vi "Logging_Example.vi"() -> ()   [LabVIEW 2024]
uses:
  Stream/Writer/DETT/DETTWriter.lvclass
  C:/Git/JA/JQMH/RQMHCore/Stream/INetworkWriter/INetworkWriter.lvclass
  LogFormatter/Default/DefaultLogFormat.lvclass
  C:/Git/JA/JQMH/RQMHCore/ErrorReporting/LogFormatter/Interface/ILogFormatter.lvclass
  LogHandle/Event/EventLogHandle.lvclass/EventLogHandle.ctl
  Record/LogRecord.lvclass/LogRecord.ctl
  RQMHLogger/Logger.lvclass/Logger.ctl
  HandleHolder/HandleHolder.lvclass/HandleHolder.ctl
  LogHandle/Stream/StreamLogHandle.lvclass
  C:/Git/JA/JQMH/RQMHCore/ErrorReporting/LogHandle/Interface/LoggingHandle.lvclass
  Stream/ConsoleWriter/ConsoleWriter.lvclass
  LogHandle/SQLiteLogHandle/SQLiteLogHandle.lvclass
  LogHandle/Event/EventLogHandle.lvclass
  <vilib>/drjdpowell/SQLite Library/SQL Connection/Connection.lvclass
  Record/LogRecord.lvclass
  LogHandle/Interface/LoggingHandle.lvclass
  RQMHLogger/Logger.lvclass
  HandleHolder/HandleHolder.lvclass
  <vilib>/drjdpowell/SQLite Library/SQLite.lvlib
  <vilib>/drjdpowell/SQLite Library/SQL Connection/Open (string).vi
  <vilib>/drjdpowell/SQLite Library/SQL Connection/Execute SQL.vi
  Shared/Level.ctl
  Shared/LoggerShared.lvlib
panel:
  out "error out 2":errorcluster
  out "Result Set":string[][](table) caption="Result Set (from first statement with results)"
  in  "stop":bool
  out "error out":errorcluster
  out "Level":T1
  out "Source":string
  out "Message":string
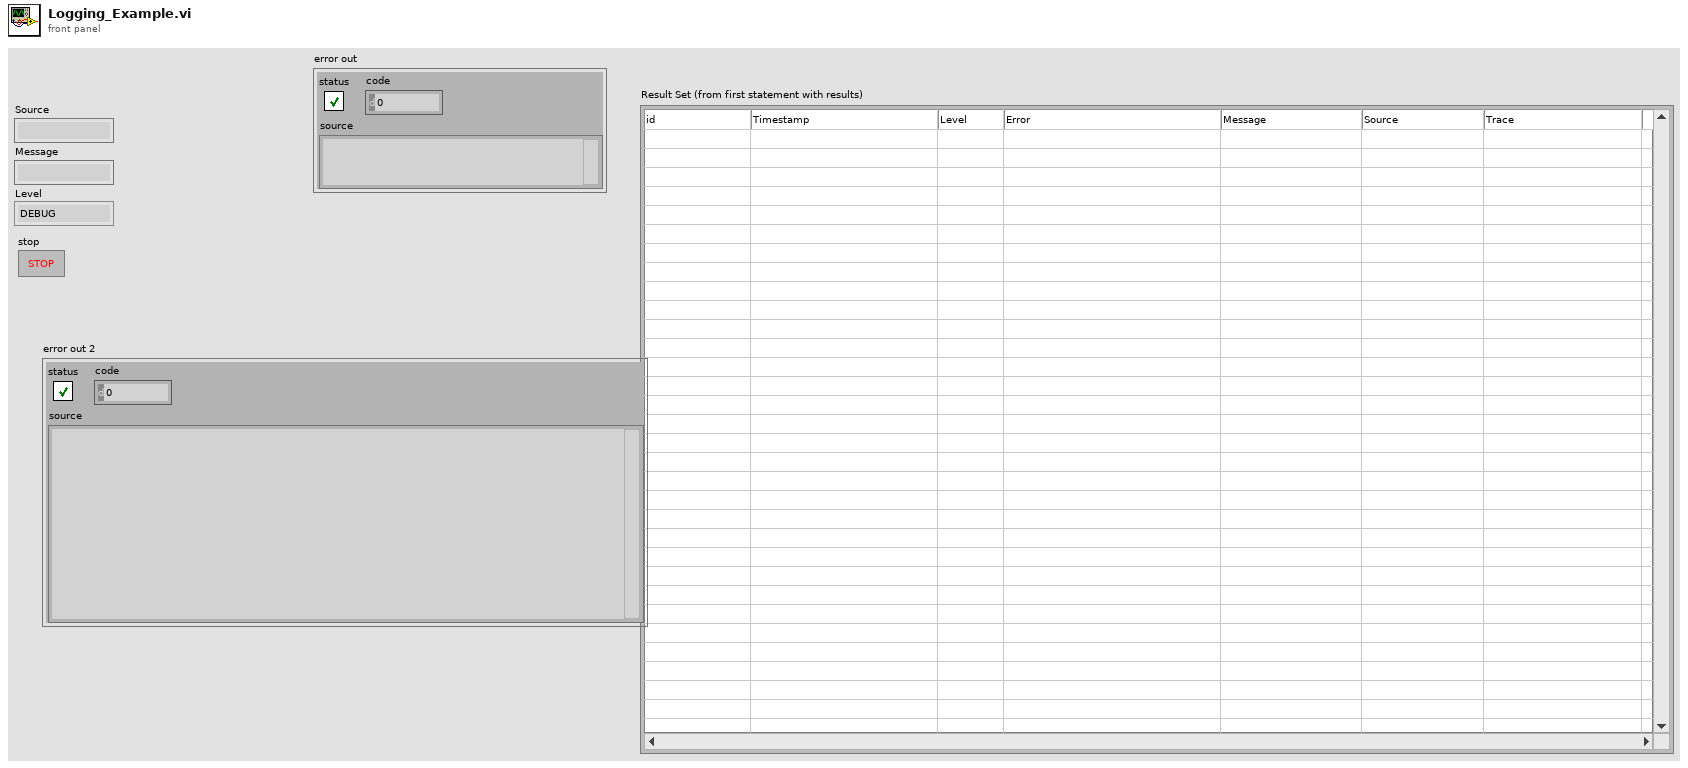
[diagram p1: front panel]
types:
  T1 = typedef "LoggerShared.lvlib/Level.ctl" = enum16{"DEBUG", "INFO", "WARNING", "ERROR", "CRITICAL"}
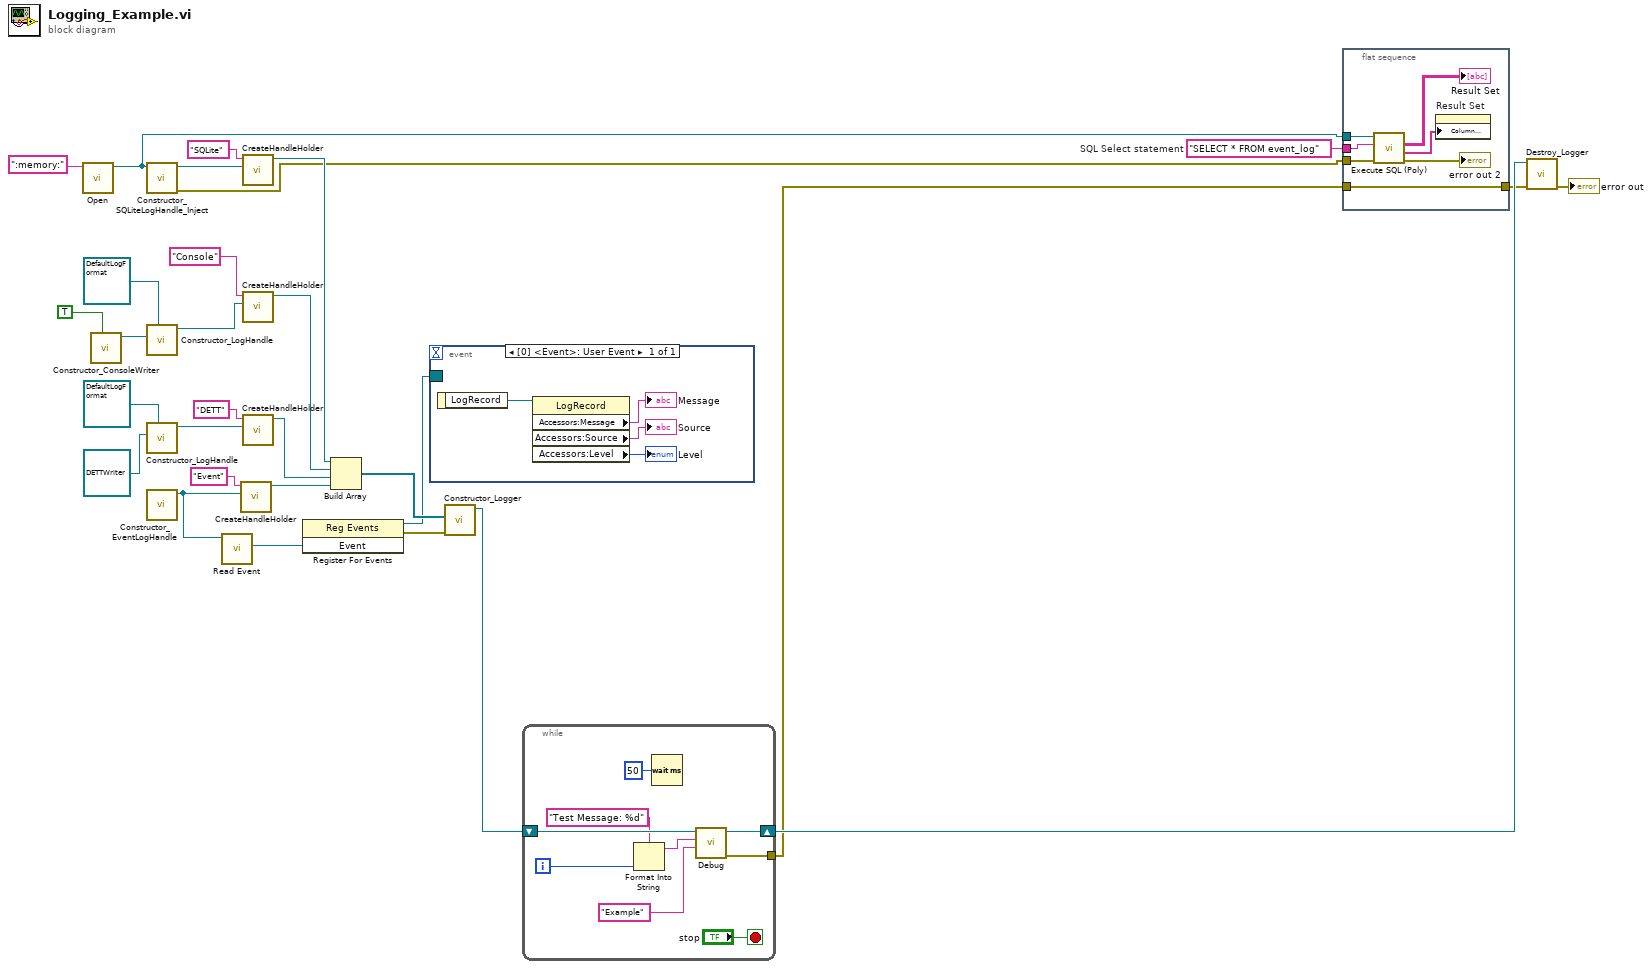
[diagram p0: block diagram]
diagram:
  w7 = "SELECT * FROM event_log"  # SQL Select statement
  (unwired) TRUE ("Autoshow? (f)")
  (unwired) refnum<class "DefaultLogFormat.lvclass"> refnum ("DefaultLogFormat.lvclass")
  n1 = call-poly <vilib>:"Open.vi"("db file"=":memory:") -> ("SQLite Connection"=w6:refnum<class "Connection.lvclass">)  [unwired: 9 in, 1 out]
  n2 = call "Constructor_ConsoleWriter.vi"("Autoshow? (f)"=TRUE) -> ("ConsoleWriter out"=w14:refnum<class "ConsoleWriter.lvclass">)  [unwired: 9 in, 1 out]
  n3 = call "Constructor_SQLiteLogHandle_Inject.vi"("Connection in"=w6) -> ("error out"=w5:errorcluster, "SQLiteLogHandle out"=w10:refnum<class "SQLiteLogHandle.lvclass">)  [unwired: 9 in]
  n4 = call "Constructor_LogHandle.vi"("Formatter"=refnum<class "DefaultLogFormat.lvclass"> refnum ("DefaultLogFormat.lvclass"), "INetworkWriter"=w14) -> ("FileHandler out"=w18:refnum<class "StreamLogHandle.lvclass">)  [unwired: 8 in, 1 out]
  n5 = call "Constructor_LogHandle.vi"("Formatter"=refnum<class "DefaultLogFormat.lvclass"> refnum ("DefaultLogFormat.lvclass"), "INetworkWriter"=refnum<class "DETTWriter.lvclass"> refnum ("DETTWriter.lvclass")) -> ("FileHandler out"=w20:refnum<class "StreamLogHandle.lvclass">)  [unwired: 8 in, 1 out]
  n6 = call "Constructor_EventLogHandle.vi"() -> ("EventHandle"=w27:refnum<class "EventLogHandle.lvclass">)  [unwired: 10 in, 1 out]
  n7 = call "Read Event.vi"("EventLogHandle in"=w27) -> ("Event"=w26:refnum<user-event>)  [unwired: 8 in, 2 out]
  n8 = call "CreateHandleHolder.vi"("Handle"=w27, "Name"="Event") -> ("HandleHolder out"=w29:refnum<class "HandleHolder.lvclass">)  [unwired: 9 in]
  n9 = call "CreateHandleHolder.vi"("Handle"=w10, "Name"="SQLite") -> ("HandleHolder out"=w8:refnum<class "HandleHolder.lvclass">)  [unwired: 9 in]
  n10 = call "CreateHandleHolder.vi"("Handle"=w18, "Name"="Console") -> ("HandleHolder out"=w15:refnum<class "HandleHolder.lvclass">)  [unwired: 9 in]
  n11 = call "CreateHandleHolder.vi"("Handle"=w20, "Name"="DETT") -> ("HandleHolder out"=w22:refnum<class "HandleHolder.lvclass">)  [unwired: 9 in]
  n12 = register-events(w26) -> (reference out=w25:refnum<event-registration>, error out=w24:errorcluster)  [unwired: 2 in]
  n13 = Build Array(w8, w15, w22, w29) -> (w28:refnum<class "HandleHolder.lvclass">[])
  n14 = event shown="[0] <Event>: User Event" {
    selector: w25 -> [_]
    dyn-events: _ -> [_]
    timeout: _ -> [_]
    event User Event {
      n15 = event-data() -> ("LogRecord"=w34:refnum<class "LogRecord.lvclass">)  [unwired: 1 in]
      n16 = property class="LogRecord"(reference=w34) -> ("Accessors:Message"=→"Message":string, "Accessors:Source"=→"Source":string, "Accessors:Level"=→"Level":T1)  [unwired: 1 in, 2 out]
    }
  }
  n17 = call "Constructor_Logger.vi"("error in (no error)"=w24, "Handles"=w28) -> ("RQMHLogger out"=w12:refnum<class "Logger.lvclass">)  [unwired: 8 in, 1 out]
  n18 = while {
    tunnel: [w40] -> w1
    shift-right: [w35] -> w4
    shift-left: w12 -> [w41]
    i -> [w37]
    stop <- "stop" stop-if-true
    n19 = Format Into String(format string="Test Message: %d" ("Message"), w37) -> (resulting string=w38:string)  [unwired: 2 in, 1 out]
    n20 = Wait (ms)(milliseconds to wait=u32 50) -> ()  [unwired: 1 out]
    n21 = call "Debug.vi"("Source"="Example", "Message"=w38, "RQMHLogger in"=w41) -> ("error out"=w40:errorcluster, "RQMHLogger out"=w35:refnum<class "Logger.lvclass">)  [unwired: 7 in]
  }
  n22 = flat-sequence {
    tunnel: w7 -> [w50]
    tunnel: w6 -> [w49]
    tunnel: w5 -> [w48]
    tunnel: [w44] -> w2
    tunnel: w1 -> [w44]
    frame #0 {
      n23 = call-poly <vilib>:"Execute SQL (Poly).vi"("error in (no error)"=w48, "SQL"=w50, "SQLite Connection in"=w49) -> ("error out"=→"error out 2":errorcluster, "Column Names"=w46:string[], "Result Set"=→"Result Set":string[][])  [unwired: 5 in, 1 out]
      n24 = property on="Result Set" class="Tbl (strict)"("Column Headers[]"=w46) -> ()  [unwired: 2 in, 2 out]
    }
  }
  n25 = call "Destroy_Logger.vi"("error in (no error)"=w2, "RQMHLogger in"=w4) -> ("error out"=→"error out":errorcluster)  [unwired: 9 in]
